vi "Unlock XNode Template.vi"(6 "error in":errorcluster, 7 "VI Ref":refnum<vi>) -> (2 "error out":errorcluster, 3 "dup VI Ref":refnum<vi>)   [LabVIEW 2025, in "XNode Support.lvlib"]
uses:
  XNode Support.lvlib
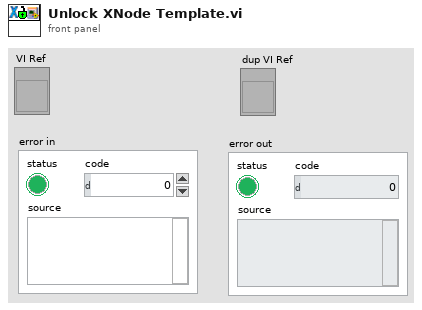
[diagram p1: front panel]
types:
  T1 = enum32{"invalid lock state", "Not Locked", "Locked (No Password)", "Password-protected"}
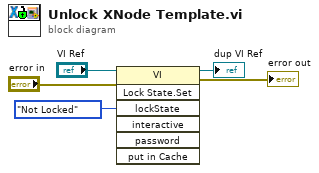
[diagram p0: block diagram]
diagram:
  n1 = invoke class="VI" method="Lock State.Set"(reference="VI Ref", error in="error in", "lockState"=T1."Not Locked" ("Lock State")) -> (reference out=→"dup VI Ref":refnum<vi>, error out=→"error out":errorcluster)  [unwired: 4 in, 5 out]
